vi "bd_terminal_label_position.vi"(8 "error in (no error)":errorcluster, 11 "VI Ref In":refnum<vi>) -> (0 "error out":errorcluster, 3 "VI Ref Out":refnum<vi>)   [LabVIEW 2018]
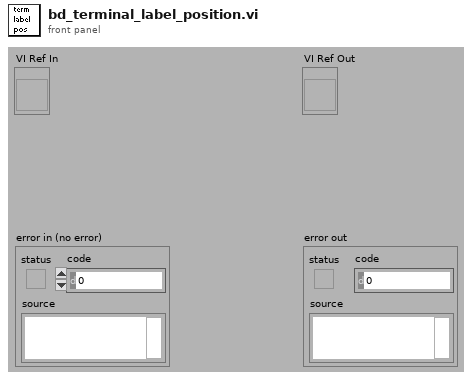
[diagram p1: front panel]
types:
  T1 = typedef "LVRectTypeDef.ctl" = cluster{"Left":i16, "Top":i16, "Right":i16, "Bottom":i16}
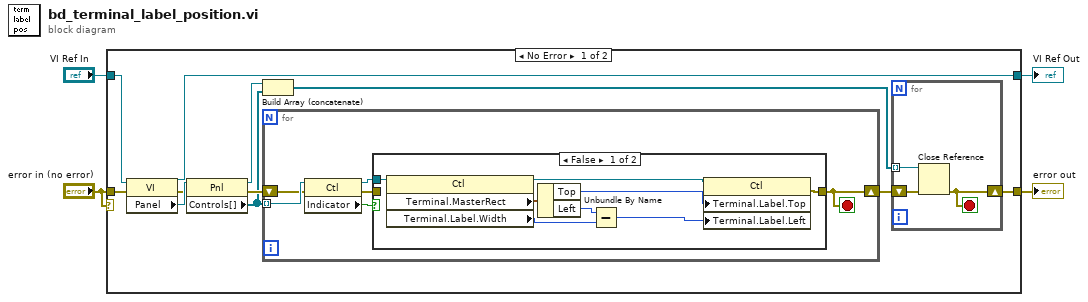
[diagram p0: block diagram]
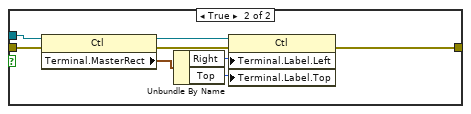
[diagram p2: hidden frame]
diagram:
  n1 = case shown="No Error" "error in (no error)" {
    tunnel: [w8 w42] -> w4
    tunnel: "VI Ref In" -> [w7 w42]
    tunnel: "error in (no error)" -> [w6 w41]
    tunnel: [w5 w41] -> w2
    frame No Error {
      n2 = property class="VI"(reference=w7, error in=w6) -> (reference out=w8:refnum<vi>, error out=w14:errorcluster, "Panel"=w15:refnum<vi>)
      n3 = property class="Pnl"(reference=w15, error in=w14) -> (reference out=w12:refnum<vi>, error out=w13:errorcluster, "Controls[]"=w11:refnum<vi>[])
      n4 = Build Array (concatenate)(w12, w11) -> (w10:refnum<vi>[])
      n5 = for {
        tunnel: w11 -> [w24] mode=indexing
        shift-right: [w19] -> w9
        shift-left: w13 -> [w21]
        stop <- w19 stop-if-true
        n6 = property class="Ctl"(reference=w24, error in=w21) -> (reference out=w23:refnum<vi>, error out=w20:errorcluster, "Indicator"=w22:bool)
        n7 = case shown="False" w22 {
          tunnel: w23 -> [w29 w38]
          tunnel: w20 -> [_ w35]
          tunnel: [w25 w33] -> w19
          frame False {
            n8 = property class="Ctl"(reference=w29) -> (reference out=w30:refnum<vi>, "Terminal.MasterRect"=w32:T1, "Terminal.Label.Width"=w31:u32)  [unwired: 1 in, 1 out]
            n9 = Unbundle By Name(w32) -> ("Top"=w28:i16, "Left"=w27:i16)
            n10 = Subtract(x=w27, y=w31) -> (x-y=w26:u32)
            n11 = property class="Ctl"(reference=w30, "Terminal.Label.Top"=w28, "Terminal.Label.Left"=w26) -> (error out=w25:errorcluster)  [unwired: 1 in, 1 out]
          }
          frame True {
            n12 = property class="Ctl"(reference=w38, error in=w35) -> (reference out=w39:refnum<vi>, error out=w34:errorcluster, "Terminal.MasterRect"=w40:T1)
            n13 = Unbundle By Name(w40) -> ("Right"=w37:i16, "Top"=w36:i16)
            n14 = property class="Ctl"(reference=w39, error in=w34, "Terminal.Label.Left"=w37, "Terminal.Label.Top"=w36) -> (error out=w33:errorcluster)  [unwired: 1 out]
          }
        }
      }
      n15 = for {
        tunnel: w10 -> [w18] mode=indexing
        shift-right: [w16] -> w5
        shift-left: w9 -> [w17]
        stop <- w16 stop-if-true
        n16 = Close Reference(reference=w18, error in (no error)=w17) -> (error out=w16:errorcluster)
      }
    }
    frame Error {
    }
  }
  "VI Ref Out" <- w4
  "error out" <- w2
